vi "Partition_Sort_Reorder.vi"(9 "Freeze Idx / Part Array":i32[](array[numeric]), 10 "Freeze / Part Array":bool[](array[boolean]), 11 "FreezeTemps / Part Array":dbl[](array[numeric])) -> (2 "Sorted Freeze Idx / Part > idx":i32[](array[numeric]), 3 "Sorted Freeze / Part > idx":dbl[][](array[numeric]))   [LabVIEW 2024]
uses:
  861c951f-c5dc-46c0-af3f-13ce072ce99f.vi
  5580c247-8882-4805-95a5-35f1be8f2dae.vi
  87b2a3f7-2712-4d38-8e39-58091931694e.vi
  <vilib>/Comparison/Less/Less Functor/Less Functor.lvclass
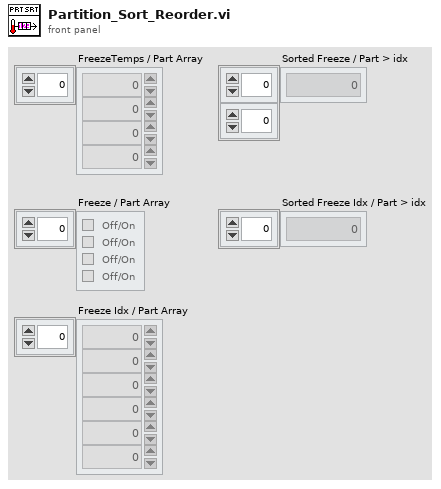
[diagram p1: front panel]
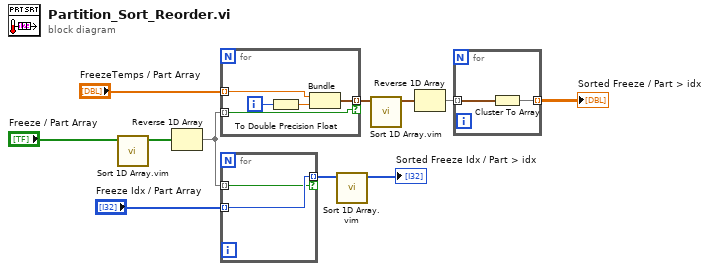
[diagram p0: block diagram]
diagram:
  n1 = call "Sort 1D Array.vim"("unsorted array"="Freeze / Part Array") -> ("sorted array"=w7:bool[])  [unwired: 10 in]
  n2 = Reverse 1D Array(array=w7) -> (reversed array=w10:bool[])
  n3 = for {
    tunnel: "FreezeTemps / Part Array" -> [w16] mode=indexing
    tunnel: [w14] -> w3 mode=indexing if=w13
    tunnel: w10 -> [w13] mode=indexing
    i -> [w15]
    n4 = To Double Precision Float(number=w15) -> (double precision float=w12:dbl)
    n5 = Bundle("Numeric"=w16, w12) -> (w14:cluster{"Numeric":dbl, dbl})  [unwired: 1 in]
  }
  n6 = for {
    tunnel: "Freeze Idx / Part Array" -> [w18] mode=indexing
    tunnel: [w18] -> w8 mode=indexing if=w17
    tunnel: w10 -> [w17] mode=indexing
  }
  n7 = call "Sort 1D Array.vim"("unsorted array"=w8) -> ("sorted array"=→"Sorted Freeze Idx / Part > idx":i32[])  [unwired: 10 in]
  n8 = call "Sort 1D Array.vim"("unsorted array"=w3) -> ("sorted array"=w4:cluster{"Numeric":dbl, dbl}[])  [unwired: 10 in]
  n9 = Reverse 1D Array(array=w4) -> (reversed array=w1:cluster{"Numeric":dbl, dbl}[])
  n10 = for {
    tunnel: w1 -> [w20] mode=indexing
    tunnel: [w19] -> w5 mode=indexing
    n11 = Cluster To Array(cluster=w20) -> (array=w19:dbl[])
  }
  "Sorted Freeze / Part > idx" <- w5
